vi "Abort Move.vi"(0 "Notifier Name In":string, 11 "Error In":errorcluster) -> (4 "Notifier Name Out":string, 15 "Error Out":errorcluster)   [LabVIEW 2020]
uses:
  Microscopes Type Defs/Microscope Notifier.ctl
  Microscopes Type Defs/Microscope Actions.ctl
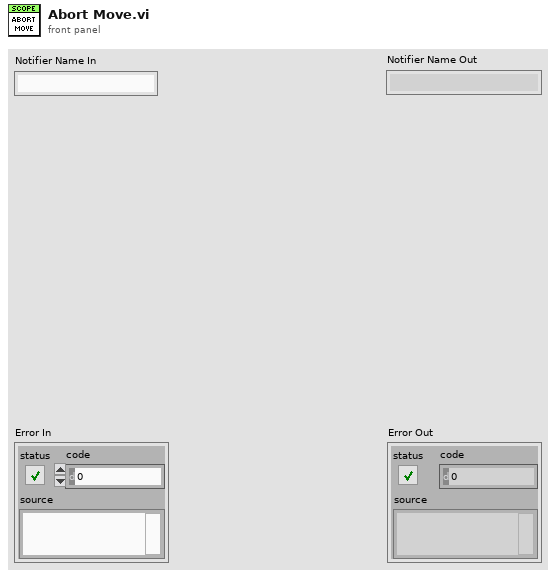
[diagram p1: front panel]
types:
  T1 = typedef "Microscope Notifier.ctl" = cluster{"Actions":T2, "Action Done":bool, "Objective Index":u8, "Objective Z Position (um)":dbl, "Lamp Index":u8, "Lamp State":bool, "Output Port":u8, "Shutter Index":u8, "Shutter State":bool, "Dichroic Wheel Position":u8, "Parameter":string, "Parameter Value":string, "Base Locked?":bool, "Obj Speed":u32, "Obj Acceleration":u32, "Obj Deceleration":u32, "Lamp Power (%)":dbl}
  T2 = typedef "Microscope Actions.ctl" = enum16{"Do Nothing", "Lock Base", "Lock Focus Knob", "Get Objective Index", "Get Objective Z Position", "Get Lamp State", "Get Lamp Power", "Get Output Port", "Get Shutter State", "Get Dichroic Wheel Position", "Set Lamp Index", "Set Shutter Index", "Set Objective Z Position", "Set Lamp State", "Set Lamp Power", "Set Output Port", "Set Shutter State", "Set Dichroic Wheel Position", "Set Objective", "Abort Move", "Set Parameter", "Get Parameter", "Quit"}
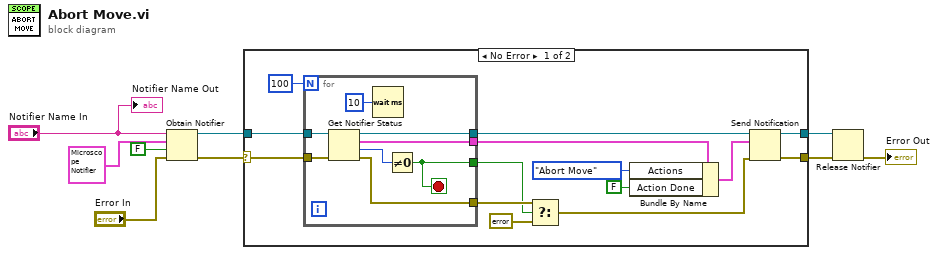
[diagram p0: block diagram]
diagram:
  n1 = Obtain Notifier(name (unnamed)="Notifier Name In", notification data type=T1 {"Actions"=enum."Get Objective Index", "Action Done"=FALSE, "Objective Index"=0, "Objective Z Position (um)"=0.0, "Lamp Index"=0, "Lamp State"=FALSE, "Output Port"=0, "Shutter Index"=0, "Shutter State"=FALSE, "Dichroic Wheel Position"=0, "Parameter"="", "Parameter Value"="", "Base Locked?"=FALSE, "Obj Speed"=0, "Obj Acceleration"=0, "Obj Deceleration"=0, "Lamp Power (%)"=0.0} ("Microscope Notifier"), create if not found? (T)=FALSE, error in (no error)="Error In") -> (notifier out=w6:refnum<notifier>, error out=w7:errorcluster)  [unwired: 1 out]
  n2 = case shown="No Error" w7 {
    selector: w7 -> [w21 w33]
    tunnel: w6 -> [w23 w32]
    tunnel: [w11 w33] -> w2
    tunnel: [w12 w32] -> w3
    frame No Error {
      n3 = for {
        N: 100 -> [_]
        tunnel: w23 -> [w31]
        tunnel: [w29] -> w13
        tunnel: [w27] -> w19
        tunnel: w21 -> [w26]
        tunnel: [w25] -> w14
        tunnel: [w24] -> w20
        stop <- w29 stop-if-true
        n4 = Get Notifier Status(notifier=w31, error in (no error)=w26) -> (notifier out=w27:refnum<notifier>, current notification=w24:T1, # waiting=w30:i32, error out=w25:errorcluster)  [unwired: 1 out]
        n5 = Wait (ms)(milliseconds to wait=u32 10) -> ()  [unwired: 1 out]
        n6 = Not Equal To 0?(x=w30) -> (x != 0?=w29:bool)
      }
      n7 = Select(t=w14, s=w13, f=errorcluster {"status"=TRUE, "code"=0, "source"="IX81 Base Error: Base busy time out."}) -> (s? t:f=w10:errorcluster)
      n8 = Bundle By Name(cluster=w20, "Actions"=Microscope_Actions."Abort Move", "Action Done"=FALSE) -> (w18:T1)
      n9 = Send Notification(notification=w18, notifier=w19, error in (no error)=w10) -> (notifier out=w12:refnum<notifier>, error out=w11:errorcluster)
    }
    frame Error {
    }
  }
  n10 = Release Notifier(notifier=w3, error in (no error)=w2) -> (error out=→"Error Out":errorcluster)  [unwired: 1 in, 2 out]
  "Notifier Name Out" <- "Notifier Name In"
